vi "XY Graph Get Scale Information.vi"(8 "error in (no error)":errorcluster, 9 "X(F)/Y(T)":bool, 10 "Plot.ScaleIdx":u32, 11 "XYGraph Ref":refnum<vi>) -> (0 "Error Out":errorcluster, 3 "Graph Scale Information":T1)   [LabVIEW 2021, in "XY Graph Add-Ons.lvlib"]
uses:
  Graph Scale Information.ctl
  XY Graph Add-Ons.lvlib
  Graphs.lvlib
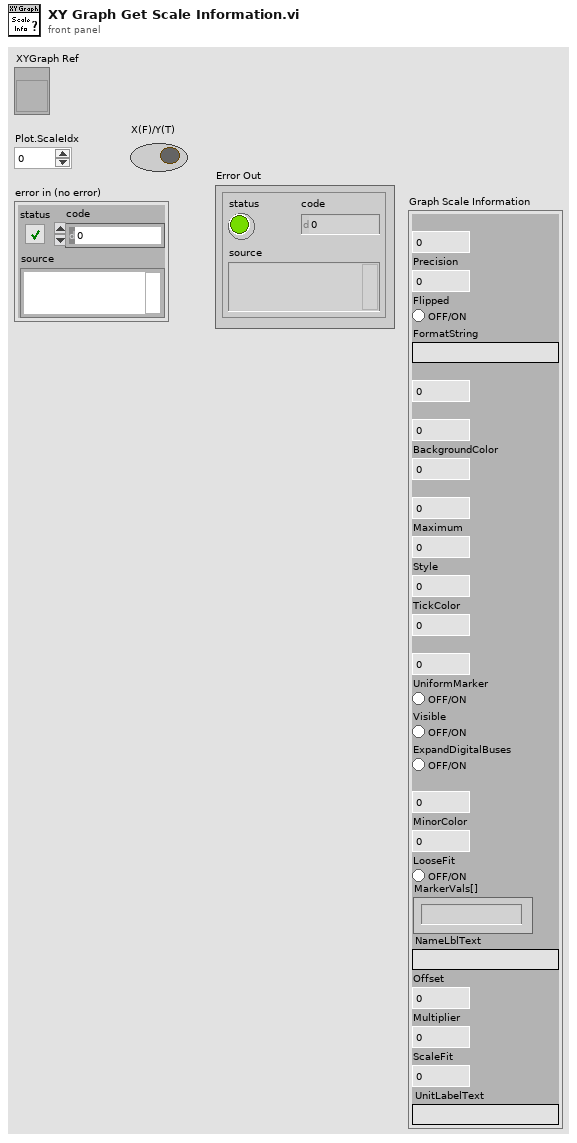
[diagram p1: front panel]
types:
  T1 = typedef "Graphs.lvlib/Graph Scale Information.ctl" = cluster{"Format":u8, "Precision":u8, "Flipped":bool, "FormatString":string, "MappingMode":u8, "TextColor":u32, "BackgroundColor":u32, "Minimum":dbl, "Maximum":dbl, "Style":u8, "TickColor":u32, "MinorTickColor":u32, "UniformMarker":bool, "Visible":bool, "ExpandDigitalBuses":bool, "MajorColor":u32, "MinorColor":u32, "LooseFit":bool, "MarkerVals[]":string, "NameLblText":string, "Offset":dbl, "Multiplier":dbl, "ScaleFit":u8, "UnitLabelText":string}
  T2 = typedef "LVFormatAndPrecisionTypeDef.ctl" = cluster{"Format":u8, "Precision":u8}
  T3 = typedef "LVTextColorsTypeDef.ctl" = cluster{"Text Color":u32, "Background Color":u32}
  T4 = typedef "LVRangeTypeDef.ctl" = cluster{"Minimum":dbl, "Maximum":dbl, "Increment":dbl, "Minor Increment":dbl, "Start":dbl}
  T5 = typedef "LVTickColorsTypeDef.ctl" = cluster{"Tick Color":u32, "Minor Tick Color":u32}
  T6 = typedef "LVMajorAndMinorColorsTypeDef.ctl" = cluster{"Major Color":u32, "Minor Color":u32}
  T7 = typedef "LVOffsetAndMultiplierTypeDef.ctl" = cluster{"Offset":dbl, "Multiplier":dbl}
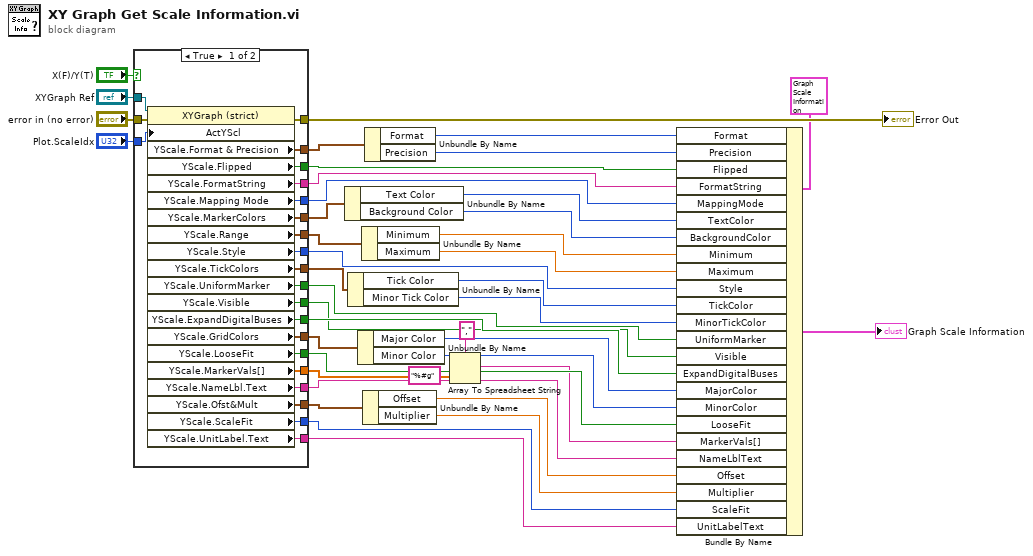
[diagram p0: block diagram]
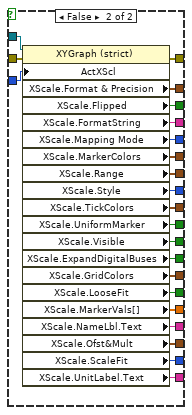
[diagram p2: hidden frame]
diagram:
  n1 = case shown="True" "X(F)/Y(T)" {
    tunnel: "error in (no error)" -> [w62 w84]
    tunnel: "Plot.ScaleIdx" -> [w61 w83]
    tunnel: "XYGraph Ref" -> [w60 w82]
    tunnel: [w59 w81] -> w37
    tunnel: [w58 w80] -> w36
    tunnel: [w57 w79] -> w35
    tunnel: [w56 w78] -> w34
    tunnel: [w55 w77] -> w33
    tunnel: [w54 w76] -> w32
    tunnel: [w53 w75] -> w31
    tunnel: [w52 w74] -> w30
    tunnel: [w51 w73] -> w2
    tunnel: [w50 w72] -> w1
    tunnel: [w49 w71] -> w3
    tunnel: [w48 w70] -> w29
    tunnel: [w47 w69] -> w28
    tunnel: [w46 w68] -> w27
    tunnel: [w45 w67] -> w26
    tunnel: [w44 w66] -> w25
    tunnel: [w43 w65] -> w24
    tunnel: [w42 w64] -> w23
    tunnel: [w41 w63] -> w22
    frame True {
      n2 = property class="XYGraph (strict)"(reference=w60, error in=w62, "ActYScl"=w61) -> (error out=w41:errorcluster, "YScale.Format & Precision"=w59:T2, "YScale.Flipped"=w58:bool, "YScale.FormatString"=w57:string, "YScale.Mapping Mode"=w56:u8, "YScale.MarkerColors"=w55:T3, "YScale.Range"=w54:T4, "YScale.Style"=w53:u8, "YScale.TickColors"=w52:T5, "YScale.UniformMarker"=w51:bool, "YScale.Visible"=w50:bool, "YScale.ExpandDigitalBuses"=w49:bool, "YScale.GridColors"=w48:T6, "YScale.LooseFit"=w47:bool, "YScale.MarkerVals[]"=w46:dbl[], "YScale.NameLbl.Text"=w45:string, "YScale.Ofst&Mult"=w44:T7, "YScale.ScaleFit"=w43:u8, "YScale.UnitLabel.Text"=w42:string)  [unwired: 1 out]
    }
    frame False {
      n3 = property class="XYGraph (strict)"(reference=w82, error in=w84, "ActXScl"=w83) -> (error out=w63:errorcluster, "XScale.Format & Precision"=w81:T2, "XScale.Flipped"=w80:bool, "XScale.FormatString"=w79:string, "XScale.Mapping Mode"=w78:u8, "XScale.MarkerColors"=w77:T3, "XScale.Range"=w76:T4, "XScale.Style"=w75:u8, "XScale.TickColors"=w74:T5, "XScale.UniformMarker"=w73:bool, "XScale.Visible"=w72:bool, "XScale.ExpandDigitalBuses"=w71:bool, "XScale.GridColors"=w70:T6, "XScale.LooseFit"=w69:bool, "XScale.MarkerVals[]"=w68:dbl[], "XScale.NameLbl.Text"=w67:string, "XScale.Ofst&Mult"=w66:T7, "XScale.ScaleFit"=w65:u8, "XScale.UnitLabel.Text"=w64:string)  [unwired: 1 out]
    }
  }
  "Error Out" <- w22
  n4 = Unbundle By Name(w33) -> ("Text Color"=w18:u32, "Background Color"=w17:u32)
  n5 = Unbundle By Name(w30) -> ("Tick Color"=w14:u32, "Minor Tick Color"=w13:u32)
  n6 = Unbundle By Name(w29) -> ("Major Color"=w12:u32, "Minor Color"=w11:u32)
  n7 = Unbundle By Name(w32) -> ("Minimum"=w16:dbl, "Maximum"=w15:dbl)
  n8 = Unbundle By Name(w25) -> ("Offset"=w10:dbl, "Multiplier"=w9:dbl)
  n9 = Unbundle By Name(w37) -> ("Format"=w20:u8, "Precision"=w19:u8)
  n10 = Array To Spreadsheet String(delimiter (Tab)=",", array=w27, 3:"%#g" ("format string")) -> (spreadsheet string=w7:string)
  n11 = Bundle By Name(cluster=T1 {"Format"=0, "Precision"=0, "Flipped"=FALSE, "FormatString"="", "MappingMode"=0, "TextColor"=0, "BackgroundColor"=0, "Minimum"=0.0, "Maximum"=0.0, "Style"=0, "TickColor"=0, "MinorTickColor"=0, "UniformMarker"=FALSE, "Visible"=FALSE, "ExpandDigitalBuses"=FALSE, "MajorColor"=0, "MinorColor"=0, "LooseFit"=FALSE, "MarkerVals[]"="", "NameLblText"="", "Offset"=0.0, "Multiplier"=0.0, "ScaleFit"=0, "UnitLabelText"=""} ("Graph Scale Information"), "Format"=w20, "Precision"=w19, "Flipped"=w36, "FormatString"=w35, "MappingMode"=w34, "TextColor"=w18, "BackgroundColor"=w17, "Minimum"=w16, "Maximum"=w15, "Style"=w31, "TickColor"=w14, "MinorTickColor"=w13, "UniformMarker"=w2, "Visible"=w1, "ExpandDigitalBuses"=w3, "MajorColor"=w12, "MinorColor"=w11, "LooseFit"=w28, "MarkerVals[]"=w7, "NameLblText"=w26, "Offset"=w10, "Multiplier"=w9, "ScaleFit"=w24, "UnitLabelText"=w23) -> (→"Graph Scale Information":T1)
